vi "chaos crest add cu.vi"(7 "dsitems":i32, 9 "ds":T1, 10 "cuname":string, 11 "connectionHandle":u32) -> (3 "function return":u32)   [LabVIEW 2014, in "libcommon-crest.lvlib"]
doc: "Add a cu to chaos\n\nchaos_crest_add_cu(handle,#name,dataset_ ##name,sizeof(dataset_ ##name)/sizeof(chaos_ds_t));"
uses:
  libcommon-crest.lvlib
  chaos-i686-dynamic-release/lib/libcommon-crest.so
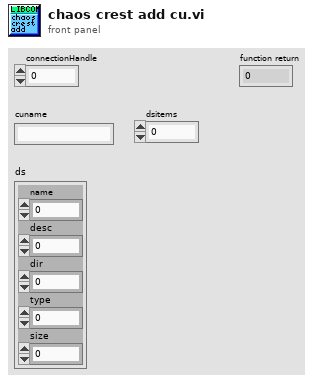
[diagram p1: front panel]
types:
  T1 = cluster{"name":u32, "desc":u32, "dir":i32, "type":i32, "size":i32}
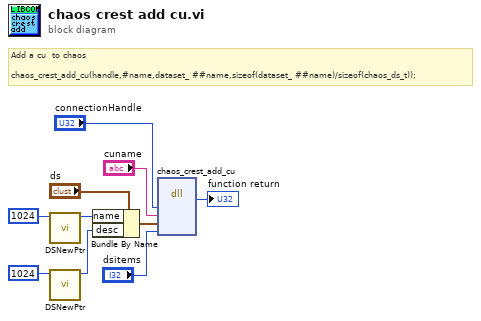
[diagram p0: block diagram]
diagram:
  # "Add a cu  to chaos\n\nchaos_crest_add_cu(handle,#name,dataset_ ##name,sizeof(dataset_ ##name)/sizeof(chaos_ds_t));"
  n1 = call <vilib>:"DSNewPtr.vi"("Size"=u64 1024) -> ("Pointer"=w4:u64)  [unwired: 9 in, 1 out]
  n2 = call <vilib>:"DSNewPtr.vi"("Size"=u64 1024) -> ("Pointer"=w2:u64)  [unwired: 9 in, 1 out]
  n3 = Bundle By Name(cluster="ds", "name"=w4, "desc"=w2) -> (w3:T1)
  n4 = dll-call lib="home/chaos/chaos_bundle/chaos-i686-dynamic-release/lib/libcommon-crest.*" fn="chaos_crest_add_cu"("connectionHandle"="connectionHandle", "cuname"="cuname", "ds"=w3, "dsitems"="dsitems") -> (→"function return":u32)  [unwired: 7 in, 2 out]
